vi "Read gestures - Leap.vi"() -> ()   [LabVIEW 2014]
panel:
  in  "Acquire":bool
  out "Finger pinch":bool[](array[boolean])
  out "Key tap":string[](array[string])=["Undetected", "Undetected", "Undetected", "Undetected", "Undetected"]
  in  "Key Tap Thresh [degree]":sgl=55.0 caption="Key Tap Threshold [degree]"
  out "Wrist Flexion/Extension":string="Undetected"
  in  "Flex Extension Thresh [degree]":sgl=45.0
  out "Palm State":string="Undetected"
  in  "Stop":bool
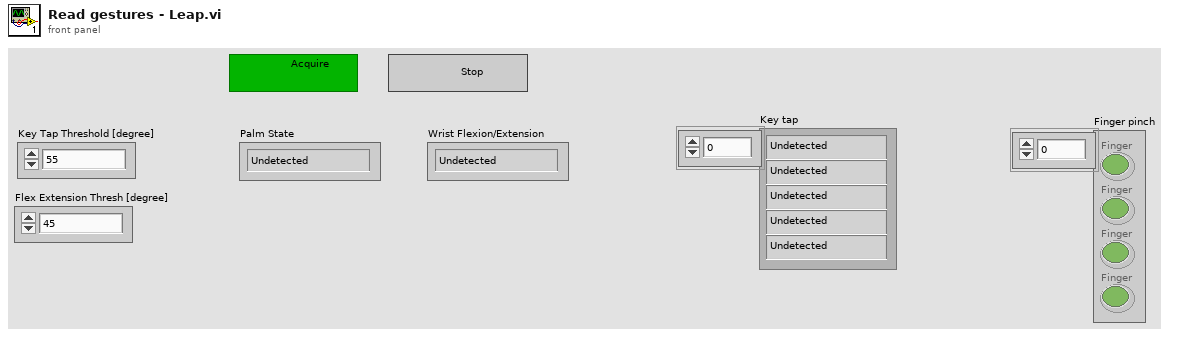
[diagram p1: front panel]
types:
  T1 = typedef "Leap Handle.ctl" = cluster{"LeapCSharp":refnum<k24>}
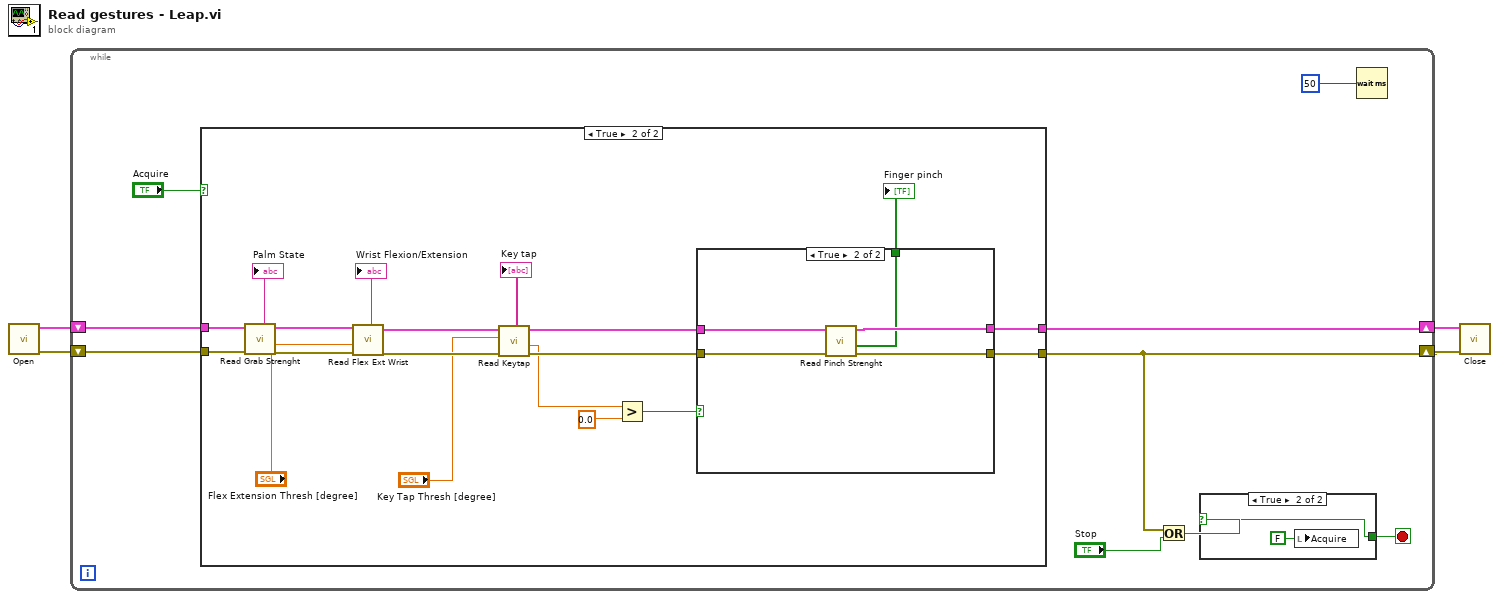
[diagram p0: block diagram]
diagram:
  n1 = call "Open.vi"() -> ("Error Out"=w3:errorcluster, "Leap Handle"=w4:T1)  [unwired: 10 in]
  n2 = while {
    shift-right: [w9] -> w2
    shift-left: w4 -> [w8]
    shift-right: [w10] -> w1
    shift-left: w3 -> [w11]
    stop <- w5 stop-if-true
    n3 = case shown="True" "Acquire" {
      tunnel: w11 -> [w17 w37]
      tunnel: [w17 w19] -> w10
      tunnel: [w18 w22] -> w9
      tunnel: w8 -> [w18 w21]
      frame False {
      }
      frame True {
        n4 = call "Read Grab Strenght.vi"("Error In"=w37, "Leap Handle In"=w21) -> ("Error Out"=w34:errorcluster, "Leap Handle Out"=w35:T1, "Palm State"=→"Palm State":string)  [unwired: 5 in, 2 out]
        n5 = call "Read Flex Ext Wrist.vi"("Error In"=w34, "Flex Extension threshold"="Flex Extension Thresh [degree]", "Leap Handle In"=w35) -> ("Error Out"=w30:errorcluster, "Wrist Flextion/Extension"=→"Wrist Flexion/Extension":string, "Leap Handle Out"=w31:T1)  [unwired: 4 in]
        n6 = call "Read Keytap.vi"("Error In"=w30, "Key Tap Thresh"="Key Tap Thresh [degree]", "Leap Handle In"=w31) -> ("Error Out"=w26:errorcluster, "PinchStrength"=w24:sgl, "Key tap"=→"Key tap":string[], "Leap Handle Out"=w27:T1)  [unwired: 3 in, 1 out]
        n7 = Greater?(x=w24, y=0.0) -> (0:w25:bool)
        n8 = case shown="True" w25 {
          tunnel: w27 -> [w39 w42]
          tunnel: w26 -> [w38 w44]
          tunnel: [w38 w43] -> w19
          tunnel: [w39 w41] -> w22
          tunnel: [_ w40] -> w23
          frame False {
          }
          frame True {
            n9 = call "Read Pinch Strenght.vi"("Error In"=w44, "Leap Handle In"=w42) -> ("Error Out"=w43:errorcluster, "Finger pinch"=w40:bool[], "Leap Handle Out"=w41:T1)  [unwired: 6 in, 1 out]
          }
        }
        "Finger pinch" <- w23
      }
    }
    n10 = Or(x=w10, y="Stop") -> (x .or. y?=w6:bool)
    n11 = case shown="True" w6 {
      selector: w6 -> [w14 w15]
      tunnel: [w14 w15] -> w5
      frame False {
      }
      frame True {
        n12 = local write "Acquire"(FALSE ("Acquire")) -> ()
      }
    }
    n13 = Wait (ms)(milliseconds to wait=u32 50) -> ()  [unwired: 1 out]
  }
  n14 = call "Close.vi"("Error In"=w1, "Leap Handle"=w2) -> ()  [unwired: 9 in, 1 out]
